vi "CRYAdd Global RcvBuffer.vi"(9 "Rcv Idx":u32, 11 "Data":i32[](array[numeric])) -> ()   [LabVIEW 2013]
uses:
  CRYMisc vis settings global.vi
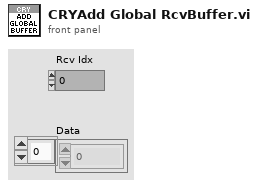
[diagram p1: front panel]
types:
  T1 = cluster{"Rcv Idx":i32, "Chn Idx":i32, "Data":i32[], "bufCount":i32}[]
  T2 = cluster{"Rcv Idx":i32, "Chn Idx":i32, "Data":i32[], "bufCount":i32}
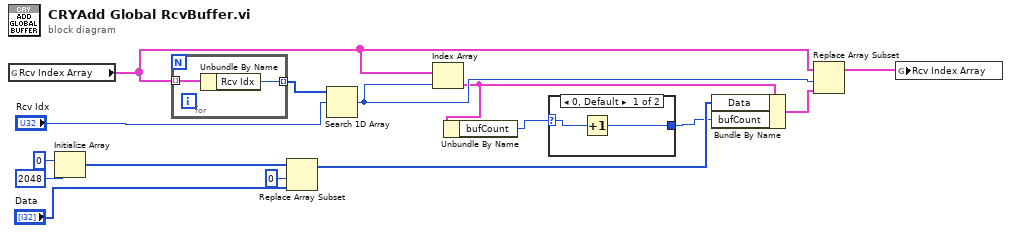
[diagram p0: block diagram]
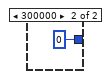
[diagram p2: hidden frame]
diagram:
  n1 = global read "CRYMisc vis settings global.vi" "Rcv Index Array"() -> (w6:T1)
  n2 = Initialize Array(0 ("element"), 2048 ("dimension size")) -> (w11:i32[])
  n3 = for {
    tunnel: w6 -> [w17] mode=indexing
    tunnel: [w16] -> w10 mode=indexing
    n4 = Unbundle By Name(w17) -> ("Rcv Idx"=w16:i32)
  }
  n5 = Replace Array Subset(array=w11, new element="Data", index=0) -> (w8:i32[])
  n6 = Search 1D Array(1D array=w10, element="Rcv Idx") -> (index of element=w5:i32)  [unwired: 1 in]
  n7 = Index Array(array=w6, index=w5) -> (element=w3:T2)
  n8 = Unbundle By Name(w3) -> ("bufCount"=w2:i32)
  n9 = case shown="0, Default" w2 {
    selector: w2 -> [w19 _]
    tunnel: [w18 0 ("bufCount")] -> w1
    frame 0, Default {
      n10 = Increment(x=w19) -> (x+1=w18:i32)
    }
    frame 300000 {
    }
  }
  n11 = Bundle By Name(cluster=w3, "Data"=w8, "bufCount"=w1) -> (w7:T2)
  n12 = Replace Array Subset(array=w6, new element=w7, index=w5) -> (w4:T1)
  n13 = global write "CRYMisc vis settings global.vi" "Rcv Index Array"(w4) -> ()
